vi "Read position in AI tasks.vi"(8 "error in (no error)":errorcluster, 11 "DAQmxTaskAIVoltage_General in":refnum<class "DAQmxTaskAIVoltage_General.lvclass">) -> (0 "error out":errorcluster, 2 "position in AI tasks":dbl, 3 "DAQmxTaskAIVoltage_General out":refnum<class "DAQmxTaskAIVoltage_General.lvclass">)   [LabVIEW 2020, in "DAQmxTaskAIVoltage_General.lvclass"]
uses:
  DAQmxTaskAIVoltage_General.lvclass
  DAQmxTaskAIVoltage_General.lvclass/DAQmxTaskAIVoltage_General.ctl
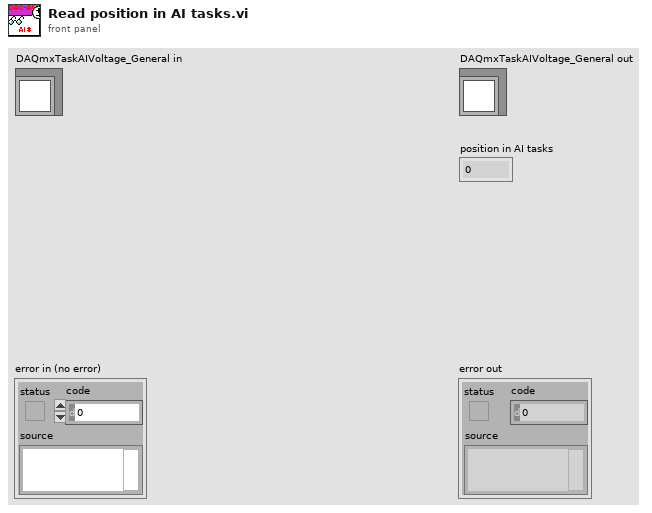
[diagram p1: front panel]
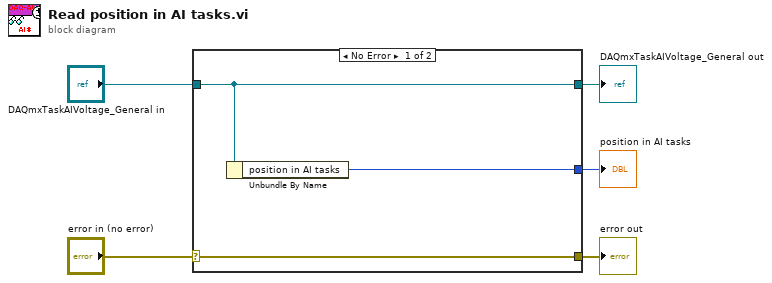
[diagram p0: block diagram]
diagram:
  n1 = case shown="No Error" "error in (no error)" {
    selector: "error in (no error)" -> [w8 w9]
    tunnel: [w8 w9] -> w4
    tunnel: [w7 w10] -> w2
    tunnel: "DAQmxTaskAIVoltage_General in" -> [w7 w10]
    tunnel: [w6 _] -> w1
    frame No Error {
      n2 = Unbundle By Name(w7) -> ("position in AI tasks"=w6:i32)
    }
    frame Error {
    }
  }
  "error out" <- w4
  "DAQmxTaskAIVoltage_General out" <- w2
  "position in AI tasks" <- w1
